vi "Helmholtz2D_Cal RHS_Difference.vi"(10 "Domain":T1={"x"={"start x"=0.0, "end x"=1.0, "# of x-points"=11}, "y"={"start y"=0.0, "end y"=1.0, "# of y-points"=11}}, 11 "X":dbl[](array[numeric])) -> (3 "Diff X":dbl[](array[numeric]))   [LabVIEW 2017, in "NI_PDE.lvlib"]
uses:
  <vilib>/gmath/NI_PDE.lvlib
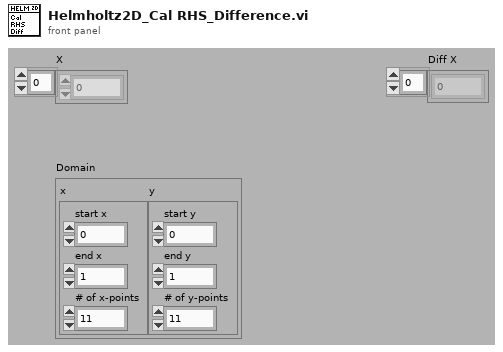
[diagram p1: front panel]
types:
  T1 = cluster{"x":cluster{"start x":dbl, "end x":dbl, "# of x-points":i32}, "y":cluster{"start y":dbl, "end y":dbl, "# of y-points":i32}}
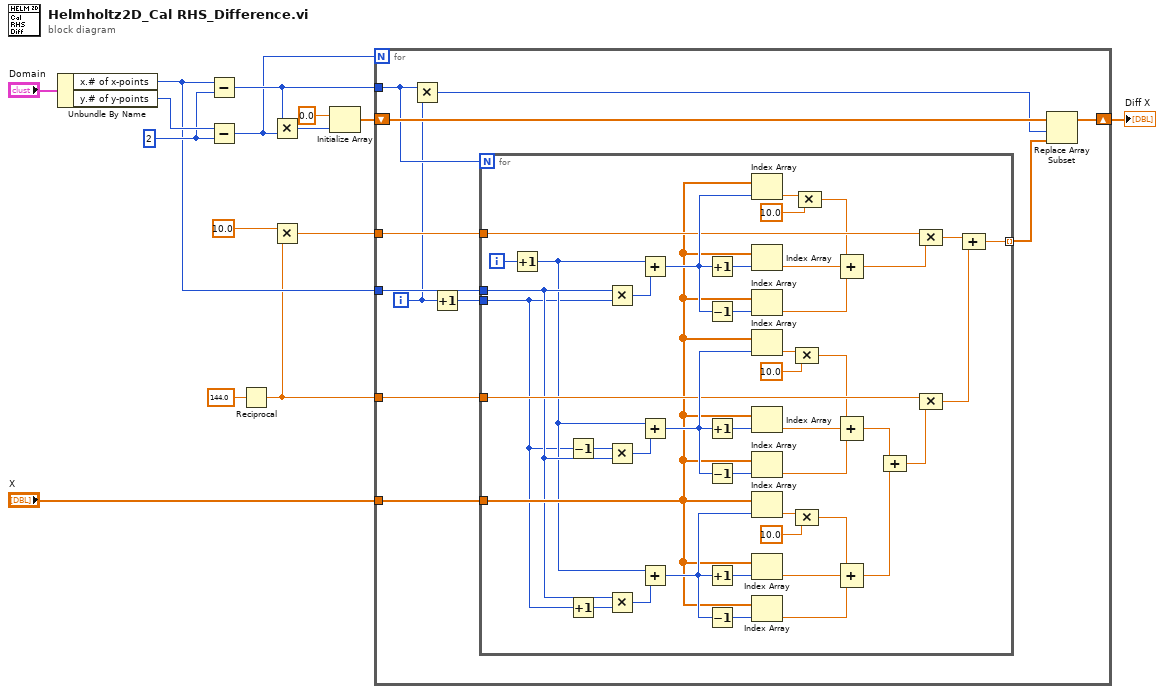
[diagram p0: block diagram]
diagram:
  w5 = 2 ("y")
  n1 = Unbundle By Name("Domain") -> ("x.# of x-points"=w3:i32, "y.# of y-points"=w6:i32)
  n2 = Subtract(x=w3, y=w5) -> (x-y=w4:i32)
  n3 = Subtract(x=w6, y=w5) -> (x-y=w2:i32)
  n4 = Reciprocal(x=144.0 ("value")) -> (1/x=w1:dbl)
  n5 = Multiply(x=w4, y=w2) -> (x*y=w9:i32)
  n6 = Multiply(x=10.0 ("value"), y=w1) -> (x*y=w12:dbl)
  n7 = Initialize Array(0.0 ("element"), w9) -> (w10:dbl[])
  n8 = for {
    N: w2 -> [_]
    tunnel: "X" -> [w24]
    tunnel: w1 -> [w25]
    tunnel: w12 -> [w26]
    tunnel: w4 -> [w18]
    tunnel: w3 -> [w22]
    shift-right: [w19] -> w8
    shift-left: w10 -> [w21]
    i -> [w16]
    n9 = Multiply(x=w18, y=w16) -> (x*y=w17:i32)
    n10 = Increment(x=w16) -> (x+1=w23:i32)
    n11 = for {
      N: w18 -> [_]
      tunnel: w23 -> [w27]
      tunnel: w26 -> [w47]
      tunnel: w25 -> [w46]
      tunnel: w24 -> [w45]
      tunnel: [w44] -> w20 mode=indexing
      tunnel: w22 -> [w29]
      i -> [w30]
      n12 = Increment(x=w30) -> (x+1=w28:i32)
      n13 = Decrement(x=w27) -> (x-1=w54:i32)
      n14 = Increment(x=w27) -> (x+1=w53:i32)
      n15 = Multiply(x=w29, y=w27) -> (x*y=w69:i32)
      n16 = Multiply(x=w54, y=w29) -> (x*y=w55:i32)
      n17 = Multiply(x=w29, y=w53) -> (x*y=w52:i32)
      n18 = Add(x=w28, y=w69) -> (x+y=w66:i32)
      n19 = Add(x=w28, y=w55) -> (x+y=w58:i32)
      n20 = Add(x=w28, y=w52) -> (x+y=w49:i32)
      n21 = Increment(x=w66) -> (x+1=w67:i32)
      n22 = Decrement(x=w66) -> (x-1=w65:i32)
      n23 = Increment(x=w58) -> (x+1=w57:i32)
      n24 = Decrement(x=w58) -> (x-1=w59:i32)
      n25 = Increment(x=w49) -> (x+1=w50:i32)
      n26 = Decrement(x=w49) -> (x-1=w48:i32)
      n27 = Index Array(array=w45, index=w66) -> (element=w68:dbl)
      n28 = Index Array(array=w45, index=w67) -> (element=w64:dbl)
      n29 = Index Array(array=w45, index=w65) -> (element=w63:dbl)
      n30 = Index Array(array=w45, index=w58) -> (element=w56:dbl)
      n31 = Index Array(array=w45, index=w57) -> (element=w60:dbl)
      n32 = Index Array(array=w45, index=w59) -> (element=w61:dbl)
      n33 = Index Array(array=w45, index=w49) -> (element=w51:dbl)
      n34 = Index Array(array=w45, index=w50) -> (element=w32:dbl)
      n35 = Index Array(array=w45, index=w48) -> (element=w31:dbl)
      n36 = Compound Arithmetic op=MULTIPLY(w56, 10.0 ("value")) -> (w38:dbl)
      n37 = Compound Arithmetic op=MULTIPLY(w51, 10.0 ("value")) -> (w36:dbl)
      n38 = Compound Arithmetic op=MULTIPLY(w68, 10.0 ("value")) -> (w42:dbl)
      n39 = Compound Arithmetic op=ADD(w42, w64, w63) -> (w62:dbl)
      n40 = Compound Arithmetic op=ADD(w38, w60, w61) -> (w35:dbl)
      n41 = Compound Arithmetic op=ADD(w36, w32, w31) -> (w34:dbl)
      n42 = Compound Arithmetic op=ADD(w35, w34) -> (w33:dbl)
      n43 = Compound Arithmetic op=MULTIPLY(w47, w62) -> (w41:dbl)
      n44 = Compound Arithmetic op=MULTIPLY(w46, w33) -> (w39:dbl)
      n45 = Compound Arithmetic op=ADD(w41, w39) -> (w44:dbl)
    }
    n46 = Replace Array Subset(array=w21, new element=w20, index=w17) -> (w19:dbl[])
  }
  "Diff X" <- w8
